vi "ContinueAcquiring.vi"(8 "error in":errorcluster, 11 "Current values":T1) -> (0 "error out":errorcluster, 3 "ContinueAcquiring?":bool)   [LabVIEW 2022 SP3, in "EClib functions.lvlib"]
uses:
  EClib functions.lvlib
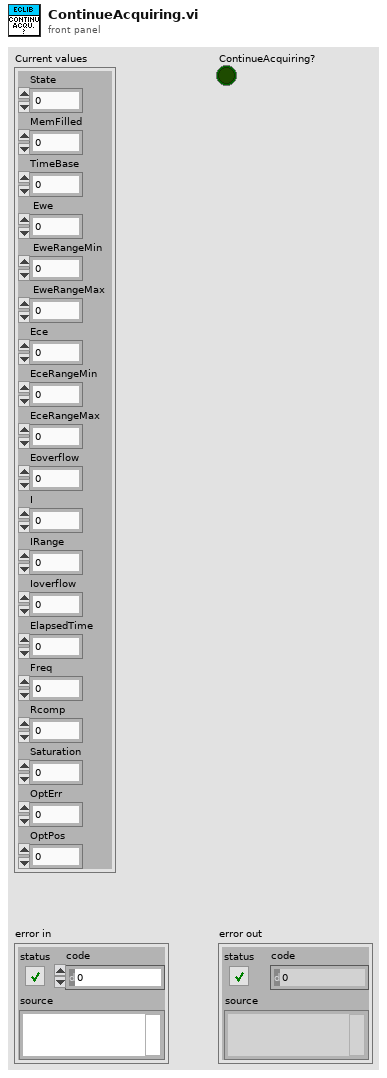
[diagram p1: front panel]
types:
  T1 = cluster{"State":i32, "MemFilled":i32, "TimeBase":sgl, " Ewe":sgl, " EweRangeMin":sgl, " EweRangeMax":sgl, "Ece":sgl, "EceRangeMin":sgl, "EceRangeMax":sgl, "Eoverflow":i32, "I":sgl, "IRange":i32, "Ioverflow":i32, "ElapsedTime":sgl, "Freq":sgl, "Rcomp":sgl, "Saturation":sgl, "OptErr":i32, "OptPos":i32}
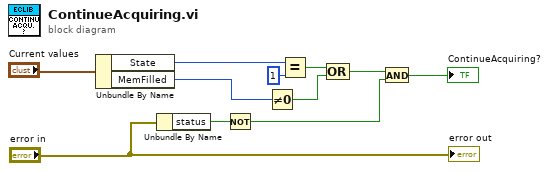
[diagram p0: block diagram]
diagram:
  n1 = Unbundle By Name("Current values") -> ("State"=w9:i32, "MemFilled"=w10:i32)
  n2 = Unbundle By Name("error in") -> ("status"=w4:bool)
  n3 = Not(x=w4) -> (.not. x?=w3:bool)
  n4 = Not Equal To 0?(x=w10) -> (x != 0?=w8:bool)
  n5 = Equal?(x=w9, y=1) -> (x = y?=w7:bool)
  n6 = Compound Arithmetic op=OR(w7, w8) -> (w2:bool)
  n7 = And(x=w2, y=w3) -> (x .and. y?=→"ContinueAcquiring?":bool)
  "error out" <- "error in"
